vi "receiveData.vi"(8 "error in (no error)":errorcluster, 11 "Controller in":refnum<class "Controller.lvclass">) -> (0 "error out":errorcluster, 2 "read buffer":string, 3 "Controller out":refnum<class "Controller.lvclass">)   [LabVIEW 2019, in "Controller.lvclass"]
uses:
  Controller.lvclass
  Controller.lvclass/Controller.ctl
  Communication/Communication.lvclass
  Axis/Axis.lvclass
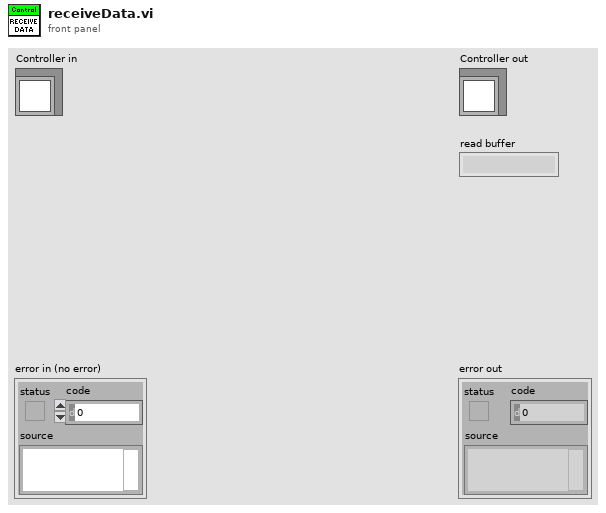
[diagram p1: front panel]
types:
  T1 = cluster{"Axes":string[], "Keys":string[], "Values":i32[]}
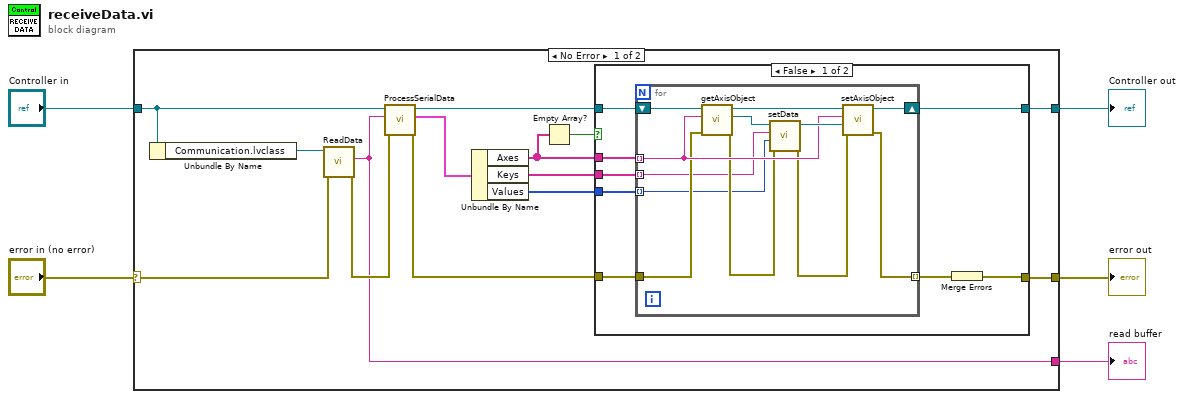
[diagram p0: block diagram]
diagram:
  n1 = case shown="No Error" "error in (no error)" {
    selector: "error in (no error)" -> [w18 w43]
    tunnel: [w17 w43] -> w4
    tunnel: [w7 w42] -> w2
    tunnel: "Controller in" -> [w15 w42]
    tunnel: [w6 _] -> w1
    frame No Error {
      n2 = Unbundle By Name(w15) -> ("Communication.lvclass"=w19:refnum<class "Communication.lvclass">)
      n3 = call-dynamic "ReadData.vi"("error in (no error)"=w18, "Communication in"=w19) -> ("error out"=w12:errorcluster, "read buffer"=w6:string)  [unwired: 7 in, 1 out]
      n4 = call "ProcessSerialData.vi"("error in (no error)"=w12, "Data in"=w6, "Controller in"=w15) -> ("error out"=w11:errorcluster, "Parsed Data"=w10:T1, "Controller out"=w16:refnum<class "Controller.lvclass">)  [unwired: 6 in]
      n5 = Unbundle By Name(w10) -> ("Axes"=w9:string[], "Keys"=w14:string[], "Values"=w13:i32[])
      n6 = Empty Array?(array=w9) -> (empty?=w8:bool)
      n7 = case shown="False" w8 {
        tunnel: [w20 w40] -> w17
        tunnel: w16 -> [w26 w41]
        tunnel: w14 -> [w25 _]
        tunnel: w13 -> [w24 _]
        tunnel: w11 -> [w23 w40]
        tunnel: w9 -> [w22 _]
        tunnel: [w21 w41] -> w7
        frame False {
          n8 = for {
            shift-right: [w35] -> w21
            shift-left: w26 -> [w38]
            tunnel: w22 -> [w34] mode=indexing
            tunnel: w25 -> [w29] mode=indexing
            tunnel: w24 -> [w28] mode=indexing
            tunnel: w23 -> [w30]
            tunnel: [w31] -> w27 mode=indexing
            n9 = call-dynamic "getAxisObject.vi"("error in (no error)"=w30, "Axis Letter"=w34, "Controller in"=w38) -> ("error out"=w33:errorcluster, "Axis Object"=w39:refnum<class "Axis.lvclass">, "Controller out"=w37:refnum<class "Controller.lvclass">)  [unwired: 6 in]
            n10 = call-dynamic "setData.vi"("error in (no error)"=w33, "Value"=w28, "Tag"=w29, "Axis in"=w39) -> ("error out"=w32:errorcluster, "Axis out"=w36:refnum<class "Axis.lvclass">)  [unwired: 6 in]
            n11 = call-dynamic "setAxisObject.vi"("error in (no error)"=w32, "Axis Object"=w36, "Axis Letter"=w34, "Controller in"=w37) -> ("error out"=w31:errorcluster, "Controller out"=w35:refnum<class "Controller.lvclass">)  [unwired: 6 in]
          }
          n12 = Merge Errors(w27) -> (w20:errorcluster)
        }
        frame True {
        }
      }
    }
    frame Error {
    }
  }
  "error out" <- w4
  "Controller out" <- w2
  "read buffer" <- w1
